vi "Initiate assembly.vi"(0 "Database Entry in":refnum<class "Database Entry.lvclass">, 11 "error in (no error)":errorcluster) -> (2 "Feet check":bool, 4 "Database Entry out":refnum<class "Database Entry.lvclass">, 6 "Module?":bool, 8 "Abort out":bool, 15 "error out":errorcluster)   [LabVIEW 2021, in "Database Entry.lvclass"]
uses:
  Database Entry.lvclass
  Database Entry.lvclass/Database Entry.ctl
  <vilib>/Utility/file.llb/Read Delimited Spreadsheet (string).vi
panel:
  out "Now assembling...":string
  in  "Abort":bool
  in  "Relative humidity":string
  in  "Temperature (C)":string
  in  "ROC version":u16(ring)=1 items=["HGCROCV3b-2", "HGCROCV3b-4", "HGCROCV3c", "Preseries"]
  in  "Adhesive":u16(ring) items=["Hybrid", "Transfer tape only", "Epoxy only"]
  in  "Module Type":u16(ring) items=["CMU,LD,Full,200,CuW", "CMU,LD,Full,300,CuW", "CMU,LD,Full,300,Ti", "CMU,LD,Full,200,CF", "CMU,LD,Full,300,CF"]
  in  "Operator":u16(ring) items=["jestein", "japicard", "simurthy", "atawker", "cmumac"]
  out "Status":dbl[][](array[numeric])
  in  "Assembly Region":cluster{"1":bool, "2":bool, "3":bool, "4":bool}
  in  "Submit":bool
  # "(To update existing modules, click 'Submit' without any selection and skip to the Manual Assembly DB.)"
  # "Tray Slot 1"
  # "Tray Slot 2"
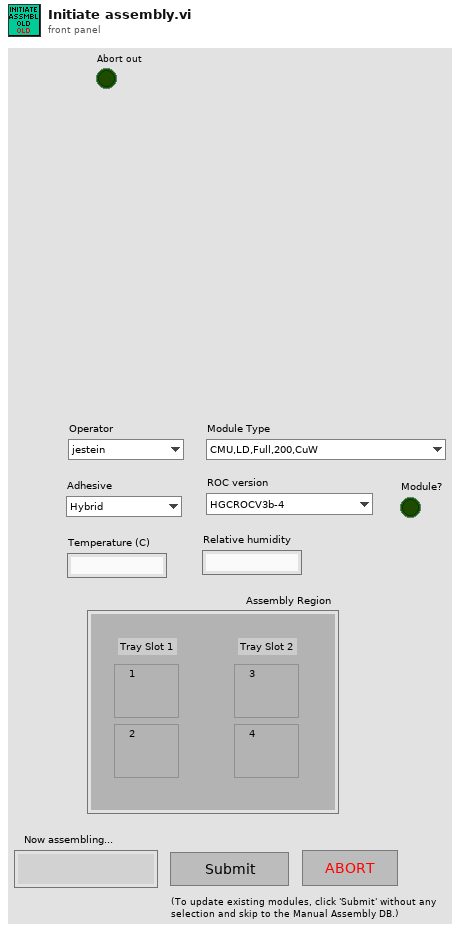
[diagram p1: front panel]
types:
  T1 = typedef "File Paths.ctl" = cluster{"Glue Pattern Folder":path, "Carrier Tray Folder":path, "Pick Up Tool Fixture Folder":path, "Components Folder":path, "Bellows Tool Offset.txt":path, "Pick Up Tool Offset.txt":path, "Dispense Tip Offset.txt":path, "Log Files":path, "Gantry Assembly Map.txt":path, "Syringe and offset map.txt":path, "Controllers Folder":path, "Local dbase config":path}
  T2 = cluster{"Temperature (C)":string, "Relative humidity":string}
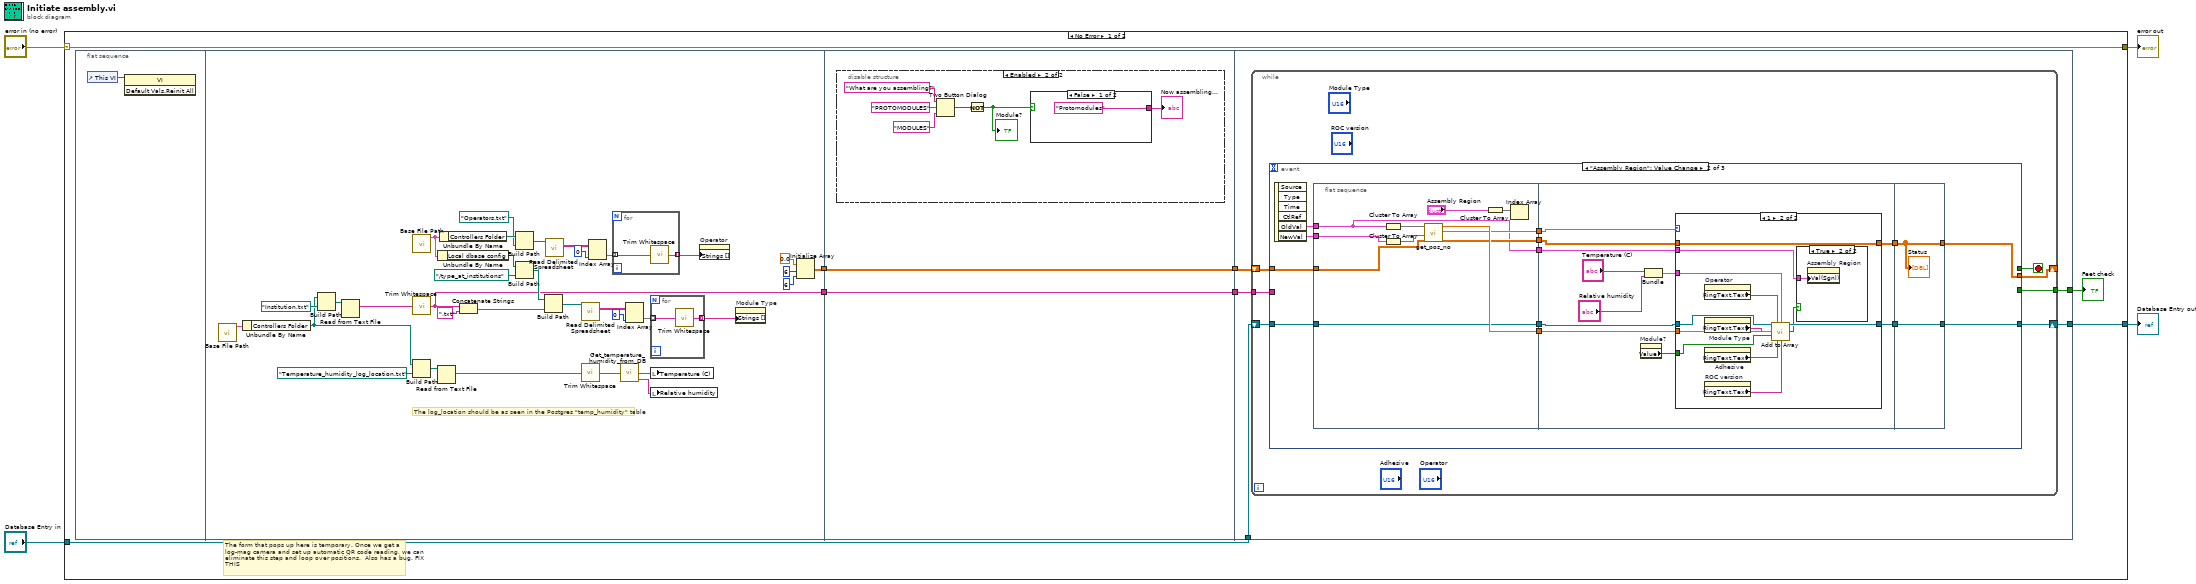
[diagram p0: block diagram]
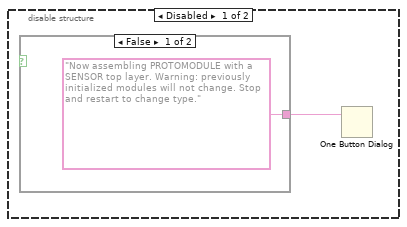
[diagram p2: hidden frame]
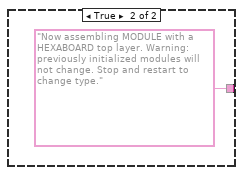
[diagram p3: hidden frame]
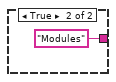
[diagram p4: hidden frame]
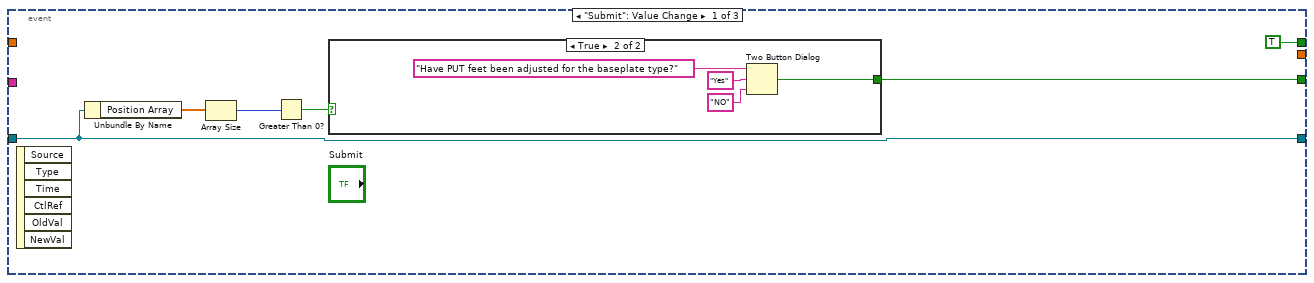
[diagram p5: hidden frame]
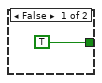
[diagram p6: hidden frame]
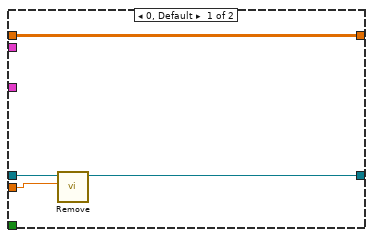
[diagram p7: hidden frame]
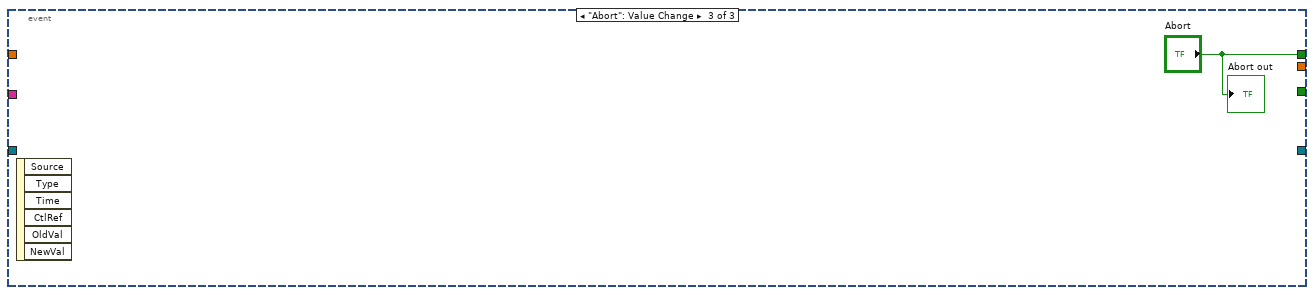
[diagram p9: hidden frame]
diagram:
  n1 = case shown="No Error" "error in (no error)" {
    selector: "error in (no error)" -> [w5 w144]
    tunnel: [w5 w144] -> w3
    tunnel: [w6 w143] -> w1
    tunnel: "Database Entry in" -> [w12 w143]
    frame No Error {
      # "The form that pops up here is temporary. Once we get a log-mag camera and set up automatic QR code reading, we can eliminate this step and loop over positions.  Also has a bug. FIX THIS"
      n2 = flat-sequence {
        tunnel: [w39] -> w10
        tunnel: [w21] -> w8
        tunnel: w10 -> [w53]
        tunnel: [w53] -> w9
        tunnel: w8 -> [w52]
        tunnel: [w52] -> w7
        tunnel: w9 -> [w68]
        tunnel: w7 -> [w67]
        tunnel: w12 -> [w69]
        tunnel: [w66] -> w6
        tunnel: [w65] -> w11
        frame #0 {
          n3 = control-ref of="This VI"() -> (w13:refnum<vi>)
          n4 = invoke class="VI" method="Default Vals.Reinit All"(reference=w13) -> ()  [unwired: 2 in, 3 out]
        }
        frame #1 {
          # "The log_location should be as seen in the Postgres \"temp_humidity\" table"
          n5 = call "Base File Path.vi"() -> ("Paths Out"=w47:T1)  [unwired: 11 in]
          n6 = Unbundle By Name(w47) -> ("Controllers Folder"=w16:path)
          n7 = Build Path(base path=w16, name or relative path=path "Institution.txt") -> (appended path=w45:path)
          n8 = Read from Text File(file (use dialog)=w45) -> (text=w22:string)  [unwired: 3 in, 3 out]
          n9 = call "Base File Path.vi"() -> ("Paths Out"=w35:T1)  [unwired: 11 in]
          n10 = call <vilib>:"Trim Whitespace.vi"("string"=w22) -> ("trimmed string"=w21:string)  [unwired: 1 in]
          n11 = Build Path(base path=w16, name or relative path=path "Temperature_humidity_log_location.txt") -> (appended path=w19:path)
          n12 = Unbundle By Name(w35) -> ("Local dbase config"=w34:path)
          n13 = Read from Text File(file (use dialog)=w19) -> (text=w18:string)  [unwired: 3 in, 3 out]
          n14 = Unbundle By Name(w35) -> ("Controllers Folder"=w44:path)
          n15 = Concatenate Strings(w21, ".txt" ("string")) -> (w28:string)
          n16 = Build Path(base path=w44, name or relative path=path "Operators.txt") -> (appended path=w42:path)
          n17 = Build Path(base path=w34, name or relative path=path "../type_at_institutions") -> (appended path=w31:path)
          n18 = Build Path(base path=w31, name or relative path=w28) -> (appended path=w30:path)
          n19 = call-poly <vilib>:"Read Delimited Spreadsheet.vi"("file path (dialog if empty)"=w42) -> ("all rows"=w41:string[][])  [unwired: 9 in, 5 out]
          n20 = call <vilib>:"Trim Whitespace.vi"("string"=w18) -> ("trimmed string"=w17:string)  [unwired: 1 in]
          n21 = call-poly <vilib>:"Read Delimited Spreadsheet.vi"("file path (dialog if empty)"=w30) -> ("all rows"=w27:string[][])  [unwired: 9 in, 5 out]
          n22 = Index Array(array=w41, index (col)=0 ("disabled index (col)")) -> (element=w26:string[])  [unwired: 1 in]
          n23 = for {
            tunnel: w26 -> [w51] mode=indexing
            tunnel: [w50] -> w25 mode=indexing
            n24 = call <vilib>:"Trim Whitespace.vi"("string"=w51) -> ("trimmed string"=w50:string)  [unwired: 1 in]
          }
          n25 = call "Get_temperature_humidity_from_DB.vi"("log_location"=w17) -> ("temp_c"=w15:string, "rel_hum"=w14:string)  [unwired: 1 out]
          n26 = Index Array(array=w27, index (col)=0 ("disabled index (col)")) -> (element=w24:string[])  [unwired: 1 in]
          n27 = for {
            tunnel: w24 -> [w49] mode=indexing
            tunnel: [w48] -> w23 mode=indexing
            n28 = call <vilib>:"Trim Whitespace.vi"("string"=w49) -> ("trimmed string"=w48:string)  [unwired: 1 in]
          }
          n29 = local write "Temperature (C)"(w15) -> ()
          n30 = local write "Relative humidity"(w14) -> ()
          n31 = property on="Operator" class="Ring (strict)"("Strings []"=w25) -> ()  [unwired: 2 in, 2 out]
          n32 = property on="Module Type" class="Ring (strict)"("Strings []"=w23) -> ()  [unwired: 2 in, 2 out]
          n33 = Initialize Array(0.0 ("element"), 6 ("dimension size"), 6 ("dimension size")) -> (w39:dbl[][])
        }
        frame #2 {
          n34 = disable-structure shown="Enabled" {
            frame Disabled {
              n35 = case shown="False" {
                selector: _ -> [_ _]
                tunnel: ["Now assembling PROTOMODULE with a SENSOR top layer. Warning: previously initialized modules will not change. Stop and restart to change type." "Now assembling MODULE with a HEXABOARD top layer. Warning: previously initialized modules will not change. Stop and restart to change type."] -> w54
                frame False {
                }
                frame True {
                }
              }
              n36 = One Button Dialog(message=w54) -> ()  [unwired: 1 in, 1 out]
            }
            frame Enabled {
              n37 = Two Button Dialog(message="What are you assembling?", 1:"MODULES" ("F button name (\"Cancel\")"), 2:"PROTOMODULES" ("T button name (\"OK\")")) -> (T button?=w59:bool)
              n38 = Not(x=w59) -> (.not. x?=w58:bool)
              "Module?" <- w58
              n39 = case shown="False" w58 {
                tunnel: ["Protomodules" ("Now assembling...") "Modules" ("Now assembling...")] -> w57
                frame False {
                }
                frame True {
                }
              }
              "Now assembling..." <- w57
            }
          }
        }
        frame #3 {
          n40 = while {
            shift-right: [w76] -> w66
            shift-left: w69 -> [w73]
            shift-right: [w74] -> _
            shift-left: w68 -> [w75]
            tunnel: w67 -> [w72]
            tunnel: [w70] -> w65
            stop <- w71 stop-if-true
            n41 = event shown="[1] \"Assembly Region\": Value Change" {
              selector: _ -> [_ _ _]
              dyn-events: _ -> [_ _ _]
              timeout: _ -> [_ _ _]
              tunnel: [TRUE ("T button?") _ "Abort"] -> w71
              tunnel: w73 -> [w80 w94 _]
              tunnel: [w80 w91 _] -> w76
              tunnel: w75 -> [_ w99 _]
              tunnel: [_ w95 _] -> w74
              tunnel: w72 -> [_ _ _]
              tunnel: [w81 _ _] -> w70
              event "Submit": Value Change {
                n42 = event-data() -> ()  [unwired: 1 in, 6 out]
                n43 = Unbundle By Name(w80) -> ("Position Array"=w79:dbl[])
                n44 = Array Size(array=w79) -> (size(s)=w78:i32)
                n45 = Greater Than 0?(x=w78) -> (x > 0?=w77:bool)
                n46 = case shown="True" w77 {
                  tunnel: [TRUE ("T button?") w84] -> w81
                  frame False {
                  }
                  frame True {
                    n47 = Two Button Dialog(message="Have PUT feet been adjusted for the baseplate type?", 1:"NO" ("F button name (\"Cancel\")"), 2:"Yes" ("T button name (\"OK\")")) -> (T button?=w84:bool)
                  }
                }
              }
              event "Assembly Region": Value Change {
                n48 = event-data() -> ("OldVal"=w88:cluster{"1":bool, "2":bool, "3":bool, "4":bool}, "NewVal"=w100:cluster{"1":bool, "2":bool, "3":bool, "4":bool})  [unwired: 1 in, 4 out]
                n49 = flat-sequence {
                  tunnel: w100 -> [w110]
                  tunnel: w88 -> [w101]
                  tunnel: w99 -> [w106]
                  tunnel: [w103] -> w97
                  tunnel: [w105] -> w96
                  tunnel: w94 -> [w104]
                  tunnel: [w104] -> w93
                  tunnel: [w102] -> w92
                  tunnel: [w101] -> w89
                  tunnel: [w121] -> w98
                  tunnel: w97 -> [w122]
                  tunnel: w96 -> [w119]
                  tunnel: w93 -> [w120]
                  tunnel: w92 -> [w118]
                  tunnel: [w117] -> w90
                  tunnel: w89 -> [w116]
                  tunnel: w98 -> [w141]
                  tunnel: [w141] -> w95
                  tunnel: [w140] -> w91
                  tunnel: w90 -> [w140]
                  frame #0 {
                    n50 = Cluster To Array(cluster=w101) -> (array=w107:bool[])
                    n51 = Cluster To Array(cluster=w110) -> (array=w108:bool[])
                    n52 = call "get_pos_no.vi"("Status Old"=w106, "Array New Status"=w108, "Array Old Status"=w107) -> ("Status New"=w103:dbl[][], "State"=w102:dbl, "Position ID"=w105:dbl)  [unwired: 2 in]
                    n53 = Cluster To Array(cluster="Assembly Region") -> (array=w111:bool[])
                    n54 = Index Array(array=w111) -> ()  [unwired: 1 in, 1 out]
                  }
                  frame #1 {
                    n55 = property on="Module?" class="Bool (strict)"() -> ("Value"=w115:bool)  [unwired: 2 in, 2 out]
                    n56 = Bundle("Temperature (C)"="Temperature (C)", "Relative humidity"="Relative humidity") -> (w112:T2)  [unwired: 1 in]
                    n57 = case shown="1" w118 {
                      tunnel: w122 -> [w123 w138]
                      tunnel: [w123 w138] -> w121
                      tunnel: w120 -> [w126 w137]
                      tunnel: [w125 w136] -> w117
                      tunnel: w119 -> [w124 w135]
                      tunnel: w115 -> [_ w134]
                      tunnel: w116 -> [_ w128]
                      tunnel: w112 -> [_ w127]
                      frame 0, Default {
                        n58 = call "Remove.vi"("Index"=w124, "Database Entry in"=w126) -> ("Database Entry out"=w125:refnum<class "Database Entry.lvclass">)  [unwired: 8 in, 1 out]
                      }
                      frame 1 {
                        n59 = property on="Operator" class="Ring (strict)"() -> ("RingText.Text"=w133:string)  [unwired: 2 in, 2 out]
                        n60 = property on="Module Type" class="Ring (strict)"() -> ("RingText.Text"=w132:string)  [unwired: 2 in, 2 out]
                        n61 = property on="Adhesive" class="Ring (strict)"() -> ("RingText.Text"=w131:string)  [unwired: 2 in, 2 out]
                        n62 = property on="ROC version" class="Ring (strict)"() -> ("RingText.Text"=w130:string)  [unwired: 2 in, 2 out]
                        n63 = call "Add to Array.vi"("Database Entry in"=w137, "Operator"=w133, "Temp and RelHumidity"=w127, "Position Index"=w135, "Module type"=w132, "Module?"=w134, "Adhesive"=w131, "ROC version"=w130) -> ("Database Entry out"=w136:refnum<class "Database Entry.lvclass">, "Position cancelled?"=w129:bool)  [unwired: 5 in, 1 out]
                        n64 = case shown="True" w129 {
                          tunnel: w128 -> [_ w139]
                          frame False {
                          }
                          frame True {
                            n65 = property on="Assembly Region" class="Clust (strict)"("Val(Sgnl)"=w139) -> ()  [unwired: 2 in, 2 out]
                          }
                        }
                      }
                    }
                  }
                  frame #2 {
                    "Status" <- w141
                  }
                }
              }
              event "Abort": Value Change {
                n66 = event-data() -> ()  [unwired: 1 in, 6 out]
                "Abort out" <- "Abort"
              }
            }
          }
        }
      }
      "Feet check" <- w11
    }
    frame Error {
    }
  }
  "error out" <- w3
  "Database Entry out" <- w1
